vi "interpolate_point.vi"(10 "x":sgl, 11 "Curve":cluster{"X":dbl[], "Y":dbl[]}) -> (3 "y":sgl)   [LabVIEW 2011]
uses:
  <vilib>/gmath/NI_Gmath.lvlib
panel:
  # "Interpolate the value at a point, given a cluster of X and Y values (as used in XY graph.)"
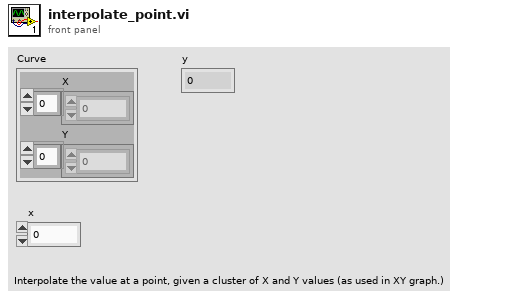
[diagram p1: front panel]
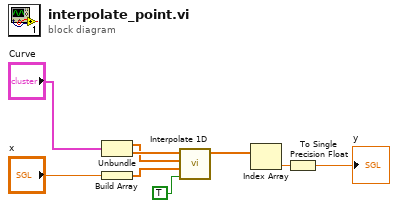
[diagram p0: block diagram]
diagram:
  n1 = Unbundle("Curve") -> ("X"=w5:dbl[], "Y"=w6:dbl[])
  n2 = Build Array("x") -> (w7:sgl[])
  n3 = call <vilib>:"Interpolate 1D.vi"("X is monotonic"=TRUE, "xi"=w7, "X"=w5, "Y"=w6) -> ("yi"=w2:dbl[])  [unwired: 5 in, 2 out]
  n4 = Index Array(array=w2) -> (element=w3:dbl)  [unwired: 1 in]
  n5 = To Single Precision Float(number=w3) -> (single precision float=→"y":sgl)
